vi "stopVoltageProtocol.vi"(2 "error in (no error)":errorcluster) -> (0 "error out":errorcluster, 1 "Error Out":u32)   [LabVIEW 2021]
uses:
  <userlib>/er4commlib_labview/er4commlib_labview.lvlib
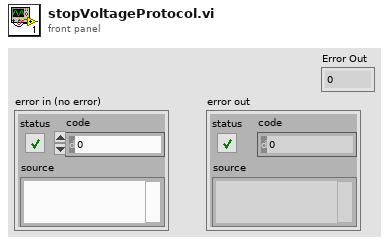
[diagram p1: front panel]
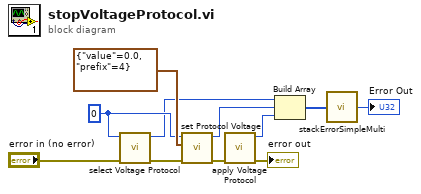
[diagram p0: block diagram]
diagram:
  w6 = u32 0 ("idx")
  n1 = call <userlib>:"select Voltage Protocol.vi"("error in (no error)"="error in (no error)", "idx"=w6) -> ("error out"=w7:errorcluster, "function return"=w5:u32)  [unwired: 8 in]
  n2 = call <userlib>:"set Protocol Voltage.vi"("error in (no error)"=w7, "voltage"=cluster{"value":dbl, "prefix":u32} {"value"=0.0, "prefix"=4} ("pulseDuration"), "idx"=w6) -> ("error out"=w8:errorcluster, "function return"=w4:u32)  [unwired: 7 in]
  n3 = call <userlib>:"apply Voltage Protocol.vi"("error in (no error)"=w8) -> ("error out"=→"error out":errorcluster, "function return"=w3:u32)  [unwired: 9 in]
  n4 = Build Array(w5, w4, w3) -> (w2:u32[])
  n5 = call "stackErrorSimpleMulti.vi"("Error List"=w2) -> ("Error Out"=→"Error Out":u32)
